vi "NamedFilesOnDrive.vi"(8 "Error In":errorcluster, 11 "Files":refnum<k24>[](array[refnum])) -> (0 "Error Out":errorcluster, 3 "Files on Drive":string[](array[string]))   [LabVIEW 2018, in "GDrive.lvlib"]
doc: "This VI outputs a list of all names of files on the User's Google Drive in an array."
uses:
  GDrive.lvlib
  Y:/UCLA Google Drive/Xavier's Retina MBP/LabVIEW/GDrive/Dependencies/Google.Apis.Drive.v3.dll
  Dependencies/Google.Apis.Drive.v3.dll
panel:
  # "This VI will create an array of file names, \nbased on the files on a given user's Google\nDrive."
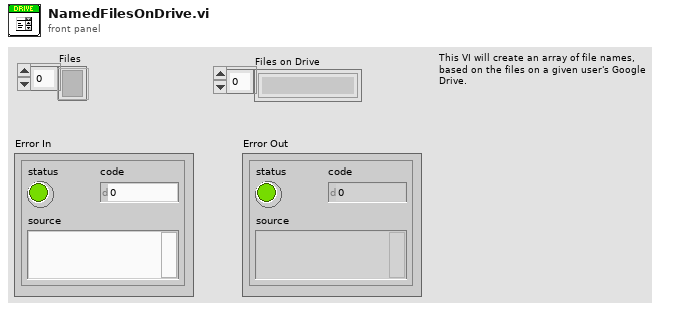
[diagram p1: front panel]
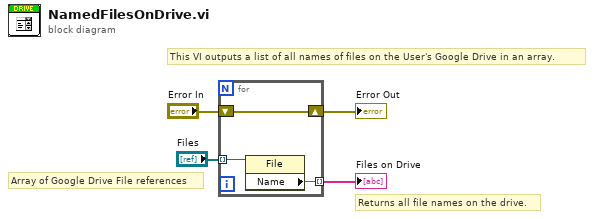
[diagram p0: block diagram]
diagram:
  # "Returns all file names on the drive."
  # "Array of Google Drive File references"
  # "This VI outputs a list of all names of files on the User's Google Drive in an array."
  n1 = for {
    tunnel: "Files" -> [w7] mode=indexing
    tunnel: [w6] -> w3 mode=indexing
    shift-right: [w5] -> w2
    shift-left: "Error In" -> [w5]
    n2 = property class="File"(reference=w7) -> ("Name"=w6:string)  [unwired: 1 in, 2 out]
  }
  "Files on Drive" <- w3
  "Error Out" <- w2
